vi "Control - GDI - Fuel Command Host.vi"() -> ()   [LabVIEW 2015, in "ECS-Host.lvlib"]
uses:
  ECS-Host.lvlib
  <vilib>/addons/Software Calibration Management/XControls/SubHost.xctl
panel:
  in  "UEGO PID":T1(xcontrol)
  out "Lambda_Des":sgl caption="[]"
  out "Fuel_FFCalc":sgl caption="[mg/cyc]"
  out "Fuel_Calc":sgl caption="[mg/cyc]"
  in  "Fuel_ManE":bool
  in  "Fuel_Man":sgl caption="[mg/cyc]"
  out "Fuel_Des":sgl caption="[mg/cyc]"
  in  "Fuel Cut":T1(xcontrol)
  # "Desired lambda setpoint"
  # "Calculated by available air \nand lambda setpoint"
  # "Modified by UEGO PID"
  # "Manual fuel per cycle"
  # "SubHosts"
  # "Final desired fuel quantity"
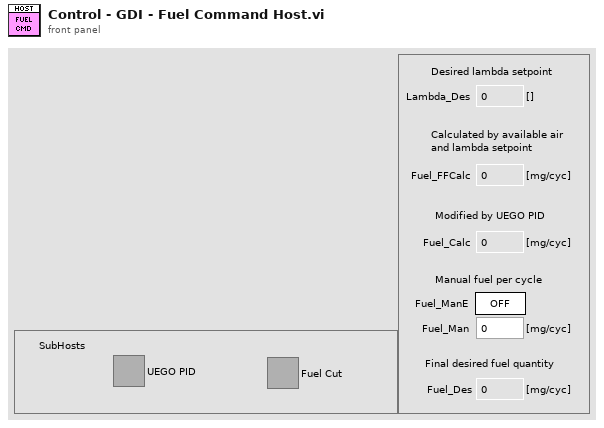
[diagram p1: front panel]
types:
  T1 = cluster{"Name":string, "Host VI":path, "Pairing File":path, "Display Name":string}
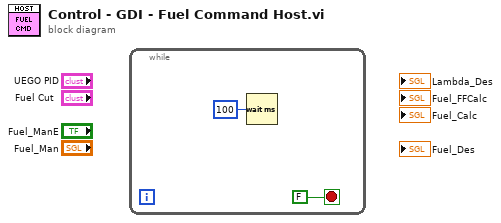
[diagram p0: block diagram]
diagram:
  n1 = while {
    stop <- FALSE stop-if-true
    n2 = Wait (ms)(milliseconds to wait=u32 100) -> ()  [unwired: 1 out]
  }
